vi "Call_signal_fromfile.vi"(6 "Plot window":string) -> (0 "Y subarray":string[](array[string]), 1 "X subarray":string[](array[string]), 2 "Curve name":string(combo), 3 "Ready?":bool)   [LabVIEW 2022 SP3]
doc: "Through this function you can select the signals stored in a CSV file."
uses:
  <vilib>/Utility/file.llb/Read Delimited Spreadsheet (string).vi
panel:
  out "Clone Name":string
  in  "Close app":bool
  in  "X data":string(combo)
  out "all rows":string[][](array[string])
  in  "Y data":string(combo)
  in  "Add":bool
  in  "Cancel":bool
  in  "From file (csv)":path caption="file path (dialog if empty)"
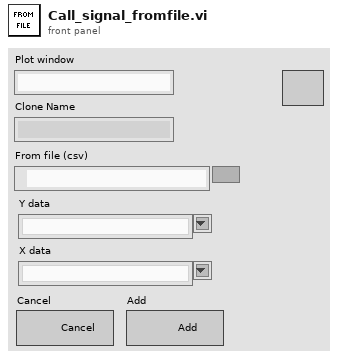
[diagram p1: front panel]
types:
  T1 = enum32{"Invalid", "Standard", "Closed", "Hidden", "Minimized", "Maximized"}
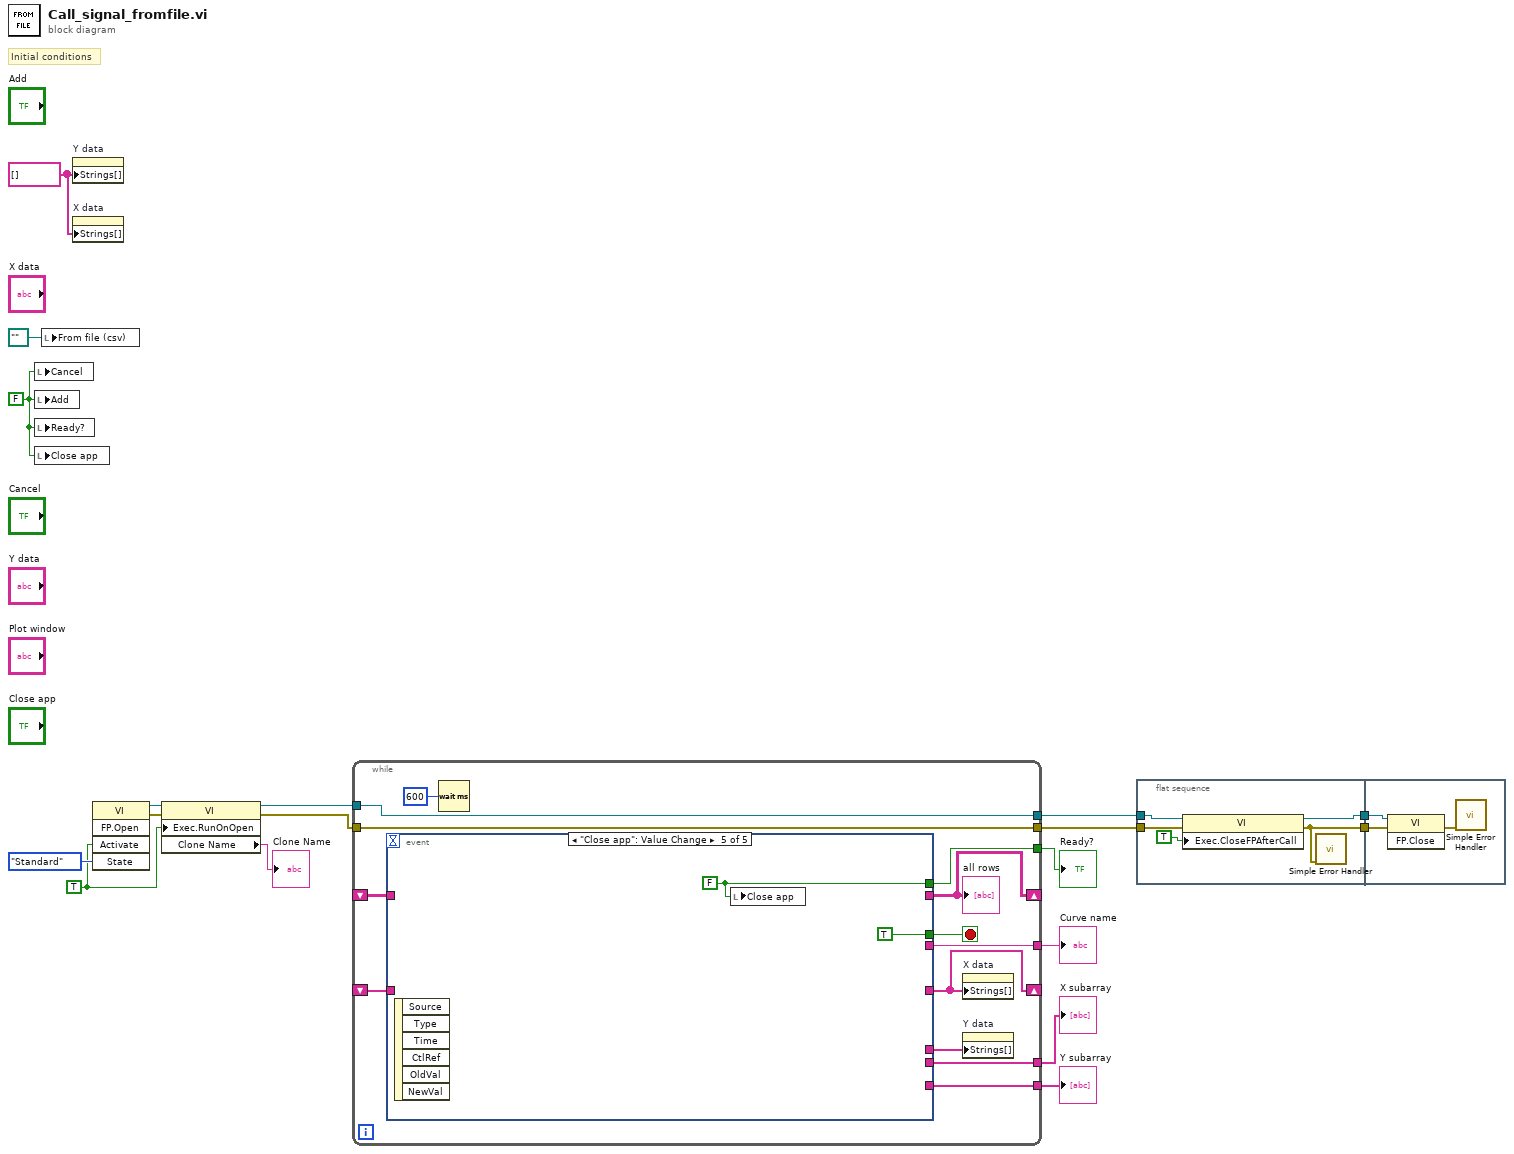
[diagram p0: block diagram]
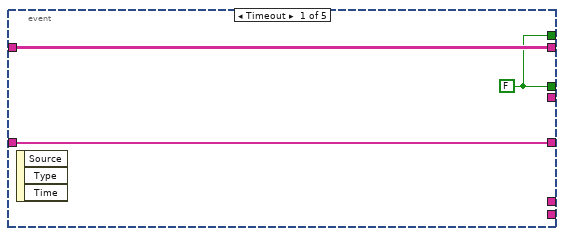
[diagram p2: hidden frame]
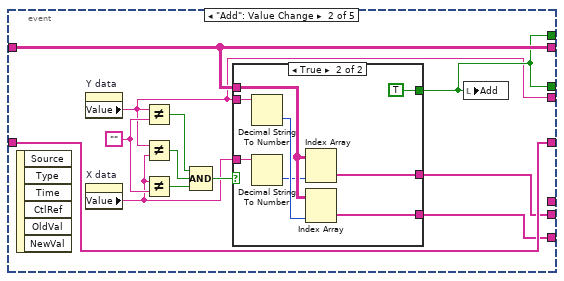
[diagram p3: hidden frame]
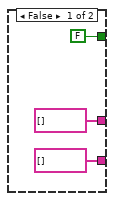
[diagram p4: hidden frame]
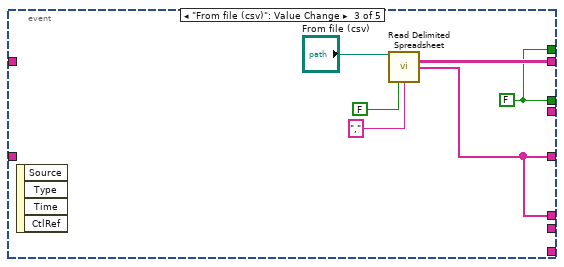
[diagram p5: hidden frame]
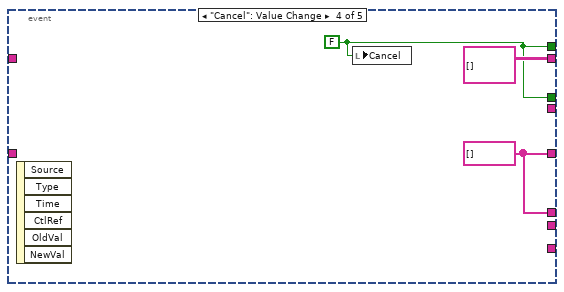
[diagram p6: hidden frame]
diagram:
  w9 = TRUE ("Activate?")
  w4 = string[] [] ("Strings []")
  w2 = FALSE
  # "Initial conditions"
  n1 = local write "Cancel"(w2) -> ()
  n2 = local write "Add"(w2) -> ()
  n3 = local write "Ready?"(w2) -> ()
  n4 = local write "Close app"(w2) -> ()
  n5 = local write "From file (csv)"(path "" ("From file (csv)")) -> ()
  n6 = property on="Y data" class="CmbBox"("Strings[]"=w4) -> ()  [unwired: 2 in, 2 out]
  n7 = property on="X data" class="CmbBox"("Strings[]"=w4) -> ()  [unwired: 2 in, 2 out]
  n8 = invoke class="VI" method="FP.Open"("Activate"=w9, "State"=T1."Standard") -> (reference out=w11:refnum<vi>, error out=w12:errorcluster)  [unwired: 3 in, 3 out]
  n9 = property class="VI"(reference=w11, error in=w12, "Exec.RunOnOpen"=w9) -> (reference out=w10:refnum<vi>, error out=w13:errorcluster, "Clone Name"=→"Clone Name":string)
  n10 = while {
    shift-right: [w28] -> _
    shift-left: _ -> [w30]
    shift-right: [w23] -> _
    shift-left: _ -> [w29]
    tunnel: [w27] -> w17
    tunnel: [w26] -> w16
    tunnel: [w24] -> w15
    tunnel: w13 -> [w21]
    tunnel: w10 -> [w22]
    tunnel: [w22] -> w8
    tunnel: [w21] -> w7
    tunnel: [w20] -> w3
    stop <- w31 stop-if-true
    n11 = event shown="[4] \"Close app\": Value Change" {
      selector: _ -> [_ _ _ _ _]
      dyn-events: _ -> [_ _ _ _ _]
      timeout: _ -> [_ _ _ _ _]
      tunnel: [w34 w41 w60 string[][] [] ("all rows") _] -> w28
      tunnel: [w33 w40 w59 w65 _] -> w23
      tunnel: [w32 w36 w58 w64 TRUE] -> w31
      tunnel: w30 -> [w34 w41 _ _ _]
      tunnel: w29 -> [w33 w40 _ _ _]
      tunnel: [_ w39 _ _ _] -> w27
      tunnel: [_ w38 _ _ _] -> w26
      tunnel: [_ _ w59 w65 _] -> w25
      tunnel: [w32 w36 w58 w64 w67] -> w24
      tunnel: [_ w35 _ _ _] -> w20
      event Timeout {
        w32 = FALSE
        n12 = event-data() -> ()  [unwired: 1 in, 3 out]
      }
      event "Add": Value Change {
        w43 = ""
        n13 = event-data() -> ()  [unwired: 1 in, 6 out]
        n14 = property on="Y data" class="CmbBox"() -> ("Value"=w35:string)  [unwired: 2 in, 2 out]
        n15 = property on="X data" class="CmbBox"() -> ("Value"=w37:string)  [unwired: 2 in, 2 out]
        n16 = Not Equal?(x=w35, y=w43) -> (x != y?=w44:bool)
        n17 = Not Equal?(x=w35, y=w37) -> (x != y?=w45:bool)
        n18 = Not Equal?(x=w37, y=w43) -> (x != y?=w46:bool)
        n19 = Compound Arithmetic op=AND(w44, w45, w46) -> (w42:bool)
        n20 = case shown="True" w42 {
          tunnel: [FALSE TRUE] -> w36
          tunnel: w41 -> [_ w54]
          tunnel: w35 -> [_ w56]
          tunnel: w37 -> [_ w53]
          tunnel: [string[] [] ("all rows") w51] -> w39
          tunnel: [string[] [] ("all rows") w50] -> w38
          frame False {
          }
          frame True {
            n21 = Decimal String To Number(string=w56) -> (number=w55:i32)  [unwired: 2 in, 1 out]
            n22 = Decimal String To Number(string=w53) -> (number=w52:i32)  [unwired: 2 in, 1 out]
            n23 = Index Array(array=w54, index (col)=w52) -> (element=w50:string[])  [unwired: 1 in]
            n24 = Index Array(array=w54, index (col)=w55) -> (element=w51:string[])  [unwired: 1 in]
          }
        }
        n25 = local write "Add"(w36) -> ()
      }
      event "From file (csv)": Value Change {
        w58 = FALSE
        n26 = event-data() -> ()  [unwired: 1 in, 4 out]
        n27 = call-poly <vilib>:"Read Delimited Spreadsheet.vi"("file path (dialog if empty)"="From file (csv)", "transpose? (F)"=FALSE, "delimiter (\\t)"="," ("delimiter (\\t)")) -> ("all rows"=w60:string[][], "first row"=w59:string[])  [unwired: 7 in, 4 out]
      }
      event "Cancel": Value Change {
        w64 = FALSE
        w65 = string[] [] ("first row")
        n28 = event-data() -> ()  [unwired: 1 in, 6 out]
        n29 = local write "Cancel"(w64) -> ()
      }
      event "Close app": Value Change {
        w67 = FALSE
        n30 = event-data() -> ()  [unwired: 1 in, 6 out]
        n31 = local write "Close app"(w67) -> ()
      }
    }
    "all rows" <- w28
    n32 = Wait (ms)(milliseconds to wait=u32 600) -> ()  [unwired: 1 out]
    n33 = property on="X data" class="CmbBox"("Strings[]"=w23) -> ()  [unwired: 2 in, 2 out]
    n34 = property on="Y data" class="CmbBox"("Strings[]"=w25) -> ()  [unwired: 2 in, 2 out]
  }
  "Y subarray" <- w17
  "X subarray" <- w16
  "Ready?" <- w15
  "Curve name" <- w3
  n35 = flat-sequence {
    tunnel: w8 -> [w73]
    tunnel: w7 -> [w72]
    tunnel: [w70] -> w6
    tunnel: [w69] -> w5
    tunnel: w6 -> [w75]
    tunnel: w5 -> [w74]
    frame #0 {
      n36 = property class="VI"(reference=w73, error in=w72, "Exec.CloseFPAfterCall"=TRUE ("Activate?")) -> (reference out=w70:refnum<vi>, error out=w69:errorcluster)
      n37 = call <vilib>:"Simple Error Handler.vi"("error in (no error)"=w69) -> ()  [unwired: 4 in, 5 out]
    }
    frame #1 {
      n38 = invoke class="VI" method="FP.Close"(reference=w75, error in=w74) -> (error out=w76:errorcluster)  [unwired: 1 in, 2 out]
      n39 = call <vilib>:"Simple Error Handler.vi"("error in (no error)"=w76) -> ()  [unwired: 4 in, 5 out]
    }
  }
